vi "Entity Table Name.vi"(10 "Entity Name":string, 11 "Database in":refnum<class "Database Platform.lvclass">) -> (2 "Table Name":string)   [LabVIEW 2022 SP3, in "Conditum.lvlib" / "Database Platform.lvclass"]
uses:
  Database Platform.lvclass
  Database Platform.lvclass/Database Platform.ctl
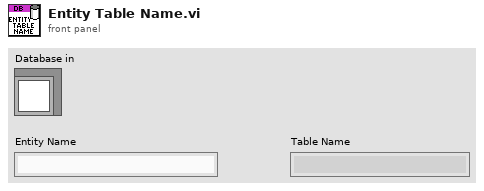
[diagram p1: front panel]
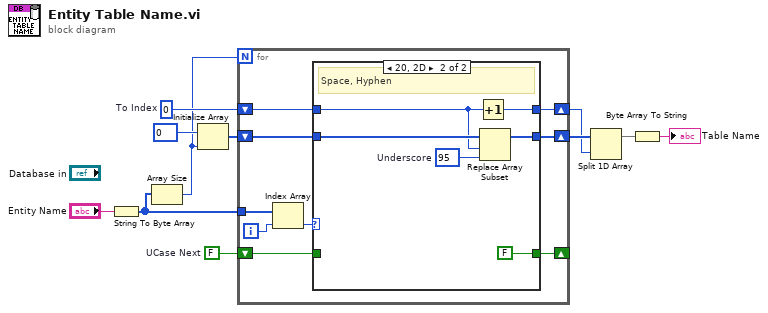
[diagram p0: block diagram]
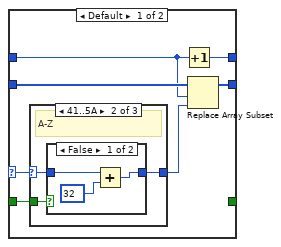
[diagram p2: hidden frame]
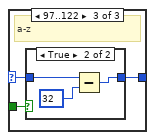
[diagram p5: hidden frame]
diagram:
  w7 = 0  # To Index
  w11 = FALSE  # UCase Next
  n1 = String To Byte Array(string="Entity Name") -> (unsigned byte array=w10:u8[])
  n2 = Array Size(array=w10) -> (size(s)=w6:i32)
  n3 = Initialize Array(u8 0, w6) -> (w8:u8[])
  n4 = for {
    N: w6 -> [_]
    tunnel: w10 -> [w20]
    shift-right: [w12] -> _
    shift-left: w11 -> [w18]
    shift-right: [w13] -> w5
    shift-left: w8 -> [w16]
    shift-right: [w14] -> w4
    shift-left: w7 -> [w17]
    i -> [w15]
    n5 = Index Array(array=w20, index=w15) -> (element=w19:u8)
    n6 = case shown="20, 2D" w19 {
      selector: w19 -> [w27 _]
      tunnel: w18 -> [w26 _]
      tunnel: w17 -> [w23 w45]
      tunnel: w16 -> [w25 w48]
      tunnel: [w22 w44] -> w14
      tunnel: [w21 w46] -> w13
      tunnel: [_ FALSE] -> w12
      frame Default {
        n7 = case shown="41..5A" w27 {
          selector: w27 -> [w28 w30 w37]
          tunnel: w26 -> [_ w31 w38]
          tunnel: [w28 w29 w36] -> w24
          frame Default {
            # "Not Letter"
          }
          frame 65..90 {
            # "A-Z"
            n8 = case shown="False" w31 {
              tunnel: w30 -> [w34 w35]
              tunnel: [w32 w35] -> w29
              frame False {
                n9 = Add(x=w34, y=u8 32) -> (x+y=w32:u8)
              }
              frame True {
              }
            }
          }
          frame 97..122 {
            # "a-z"
            n10 = case shown="True" w38 {
              tunnel: w37 -> [w39 w42]
              tunnel: [w39 w40] -> w36
              frame False {
              }
              frame True {
                n11 = Subtract(x=w42, y=u8 32) -> (x-y=w40:u8)
              }
            }
          }
        }
        n12 = Increment(x=w23) -> (x+1=w22:i32)
        n13 = Replace Array Subset(array=w25, new element=w24, index=w23) -> (w21:u8[])
      }
      frame 32, 45 {
        w43 = u8 95  # Underscore
        # "Space, Hyphen"
        n14 = Increment(x=w45) -> (x+1=w44:i32)
        n15 = Replace Array Subset(array=w48, new element=w43, index=w45) -> (w46:u8[])
      }
    }
  }
  n16 = Split 1D Array(array=w5, index=w4) -> (first subarray=w3:u8[])  [unwired: 1 out]
  n17 = Byte Array To String(unsigned byte array=w3) -> (string=→"Table Name":string)
